vi "datasocket.vi"() -> ()   [LabVIEW 2011]
panel:
  out "Numeric":dbl
  in  "stop":bool
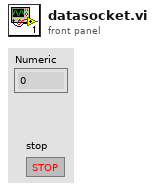
[diagram p1: front panel]
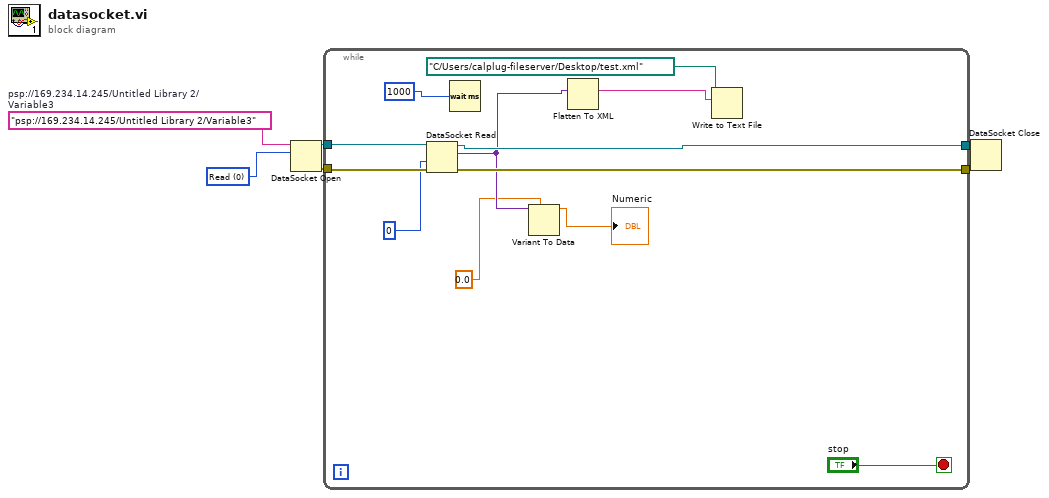
[diagram p0: block diagram]
diagram:
  w5 = u16 0 items=["Read"]
  w6 = "psp://169.234.14.245/Untitled Library 2/Variable3"  # psp://169.234.14.245/Untitled Library 2/Variable3
  n1 = DataSocket Open(10:w5, 11:w6) -> (0:w4:errorcluster, 3:w3:refnum<k13>)  [unwired: 2 in]
  n2 = while {
    tunnel: w4 -> [w15]
    tunnel: w3 -> [w16]
    tunnel: [w12] -> w2
    tunnel: [w14] -> w1
    stop <- "stop" stop-if-true
    n3 = DataSocket Read(8:w15, 9:0, 11:w16) -> (0:w12:errorcluster, 2:w9:variant, 3:w14:refnum<k13>)  [unwired: 2 in, 4 out]
    n4 = Wait (ms)(milliseconds to wait=1000) -> ()  [unwired: 1 out]
    n5 = Variant To Data(type=0.0, Variant=w9) -> (data=→"Numeric":dbl)  [unwired: 1 in, 1 out]
    n6 = Flatten To XML(anything=w9) -> (xml string=w11:string)
    n7 = Write to Text File(file (use dialog)=path "C:/Users/calplug-fileserver/Desktop/test.xml", text=w11) -> ()  [unwired: 2 in, 3 out]
  }
  n8 = DataSocket Close(8:w2, 11:w1) -> ()  [unwired: 1 in, 2 out]
